vi "Setup Serial (SubVI).vi"(11 "VISA Refnum in":refnum<visa-resource-name>) -> (0 "error out":errorcluster, 3 "VISA Refnum out":refnum<visa-resource-name>)   [LabVIEW 2019]
uses:
  <vilib>/Instr/_visa.llb/VISA Set IO Buffer Mask.ctl
  <vilib>/Instr/_visa.llb/VISA Configure Serial Port (Instr).vi
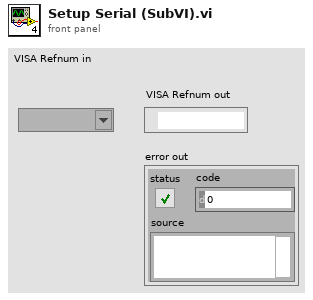
[diagram p1: front panel]
types:
  T1 = typedef "VISA Set IO Buffer Mask.ctl" = u16
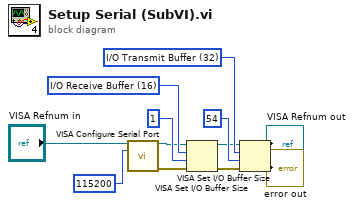
[diagram p0: block diagram]
diagram:
  w10 = T1 32 items=["I/O Receive Buffer"=16, "I/O Transmit Buffer"=32, "I/O Receive and Transmit Buffer"=48] ("Mask")
  w5 = T1 16 items=["I/O Receive Buffer"=16, "I/O Transmit Buffer"=32, "I/O Receive and Transmit Buffer"=48] ("Mask")
  n1 = call-poly "VISA Configure Serial Port"("VISA resource name"="VISA Refnum in", "baud rate (115200)"=u32 115200 ("baud rate (9600)")) -> ("VISA resource name out"=w2:refnum<visa-resource-name>, "error out"=w3:errorcluster)  [unwired: 12 in]
  n2 = VISA Set I/O Buffer Size(VISA resource name=w2, mask (16)=w5, size (4096)=u32 1, error in (no error)=w3) -> (VISA resource name out=w7:refnum<visa-resource-name>, error out=w6:errorcluster)
  n3 = VISA Set I/O Buffer Size(VISA resource name=w7, mask (16)=w10, size (4096)=u32 54, error in (no error)=w6) -> (VISA resource name out=→"VISA Refnum out":refnum<visa-resource-name>, error out=→"error out":errorcluster)
